vi "ParseMainStream.vi"(10 "Image Dst":T1, 11 "Image":T1) -> (3 "Image Out":T1)   [LabVIEW 2015]
uses:
  <vilib>/vision/Image Controls.llb/IMAQ Image.ctl
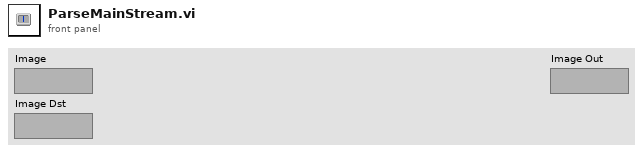
[diagram p1: front panel]
types:
  T1 = typedef "IMAQ Image.ctl" = refnum<image>
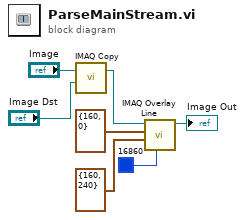
[diagram p0: block diagram]
diagram:
  n1 = call "IMAQ Copy"("Image Dst"="Image Dst", "Image Src"="Image") -> ("Image Dst Out"=w2:T1)  [unwired: 4 in, 1 out]
  n2 = call "IMAQ Overlay Line"("Color"=u32 16860, "End Point"=cluster{"X":i32, "Y":i32} {"X"=160, "Y"=240}, "Start Point"=cluster{"X":i32, "Y":i32} {"X"=160, "Y"=0}, "Image"=w2) -> ("Image Out"=→"Image Out":T1)  [unwired: 6 in, 1 out]
